vi "PIM System Warning.vi"(6 "Driver Ref (null)":T1, 8 "error in (no error)":errorcluster, 10 "PIM Test Parameters":T2={"Stimulus"={"C1 Pwr dBm"=0.0, "C2 Pwr dBm"=0.0, "Power Units"=enum."dBm", "Meas Type"=enum."Time", "C1 Freq MHz"=0.0, "C2 Freq MHz"=0.0, "Swept Freq Step"=0}, "Measure"={"IM Order"=0, "Direction"=0, "Averaging"=1, "ALC ON?"=TRUE, "Peak Hold?"=TRUE, "Peak last N"=1, "Ref Level dBm"=-100.0, "Ref Units"=enum."dBm", "Num Samples"=1, "Sample units"=enum."Sample(s)", "Update Rate (s)"=0.0, "DUT PORT"=enum."Port 1", "Percent (%)"=100}, "Display"={"Power Scale"={"yRange_min"=0, "yRange_max"=0}, "xRange_span"=5}} {"Stimulus"."Swept Freq Step" items=[".2", ".4", "1.0", "2.0"]; "Measure"."Averaging" items=["None", "Minimum", "Normal", "High", "Maximum"]; "Measure"."Direction" items=["Reverse", "Forward", "Auxiliary"]; "Measure"."IM Order" items=["3rd", "5th", "7th", "9th", "11th", "13th", "15th", "17th", "19th", "21st", "23rd", "25th", "27th", "29th", "31st", "33rd"]}, 11 "TestSetDef":T12={"General"={"ID"=0, "Model"="", "Dual Port?"=FALSE, "Options"="", "Options"={"E"=FALSE, "K"=FALSE, "H"=FALSE, "W"=FALSE, "F"=FALSE}, "Cal File"=path ""}, "Receiver"={"Fstart, MHz"=0.0, "Fstop MHz"=0.0, "Fstep MHz"=0.0, "IF, MHz"=0.0}, "RX Band"={"Fstart, MHz"=0.0, "Fstop MHz"=0.0}, "TX 1"={"Fstart, MHz"=0.0, "Fstop MHz"=0.0, "Pmax, dBm"=0.0, "Pstep, dB"=0.0}, "TX 2"={"Fstart, MHz"=0.0, "Fstop MHz"=0.0, "Pmax, dBm"=0.0, "Pstep, dB"=0.0}, "Low-side?"=TRUE}) -> (2 "Message (\"\")":string="\n\n", 3 "Abort?":bool)   [LabVIEW 2011]
uses:
  BPIMCore/HW IO/Test Set Definition.ctl
  TypeDefs/PIM Test Parameters.ctl
  TypeDefs/PIM Stimulus Parameters.ctl
  BPIMCore/HW IO/PIM Sweep Step Size.ctl
  TypeDefs/PIM Measurement Parameters.ctl
  BPIMCore/HW IO/IMOrder.ctl
  BPIMCore/HW IO/MeasMode.ctl
  BPIMCore/HW IO/HW Averaging.ctl
  TypeDefs/PIM Meas Units.ctl
  BPIMCore/HW IO/DUTport.ctl
  TypeDefs/PIM Display Parameters.ctl
  drivers/PIM/PIM Driver Ref.ctl
  drivers/PIM/PIM Command.ctl
panel:
  in  "B 2":bool
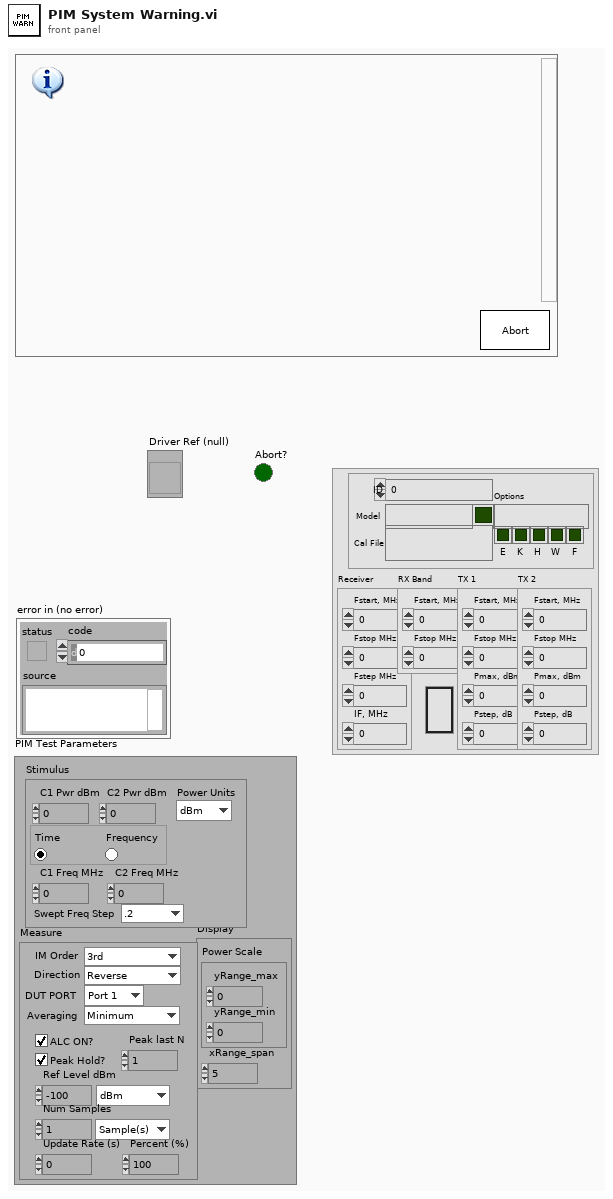
[diagram p1: front panel]
types:
  T1 = typedef "PIM Driver Ref.ctl" = refnum<vi>
  T2 = typedef "PIM Test Parameters.ctl" = cluster{"Stimulus":T3, "Measure":T5, "Display":T11}
  T3 = typedef "PIM Stimulus Parameters.ctl" = cluster{"C1 Pwr dBm":dbl, "C2 Pwr dBm":dbl, "Power Units":enum16{"dBm", "Watts"}, "Meas Type":enum32{"Time", "Frequency"}, "C1 Freq MHz":dbl, "C2 Freq MHz":dbl, "Swept Freq Step":T4}
  T4 = typedef "PIM Sweep Step Size.ctl" = u16
  T5 = typedef "PIM Measurement Parameters.ctl" = cluster{"IM Order":T6, "Direction":T7, "Averaging":T8, "ALC ON?":bool, "Peak Hold?":bool, "Peak last N":u32, "Ref Level dBm":dbl, "Ref Units":enum16{"dBm", "dBc"}, "Num Samples":u32, "Sample units":T9, "Update Rate (s)":dbl, "DUT PORT":T10, "Percent (%)":u8}
  T6 = typedef "IMOrder.ctl" = u8
  T7 = typedef "MeasMode.ctl" = u16
  T8 = typedef "HW Averaging.ctl" = u16
  T9 = typedef "PIM Meas Units.ctl" = enum16{"Sample(s)", "Second(s)", "Sweep(s)"}
  T10 = typedef "DUTport.ctl" = enum16{"Port 1", "Port 2"}
  T11 = typedef "PIM Display Parameters.ctl" = cluster{"Power Scale":cluster{"yRange_min":i32, "yRange_max":i32}, "xRange_span":u32}
  T12 = typedef "Test Set Definition.ctl" = cluster{"General":cluster{"ID":u32, "Model":string, "Dual Port?":bool, "Options":string, "Options":cluster{"E":bool, "K":bool, "H":bool, "W":bool, "F":bool}, "Cal File":path}, "Receiver":cluster{"Fstart, MHz":dbl, "Fstop MHz":dbl, "Fstep MHz":dbl, "IF, MHz":dbl}, "RX Band":cluster{"Fstart, MHz":dbl, "Fstop MHz":dbl}, "TX 1":cluster{"Fstart, MHz":dbl, "Fstop MHz":dbl, "Pmax, dBm":dbl, "Pstep, dB":dbl}, "TX 2":cluster{"Fstart, MHz":dbl, "Fstop MHz":dbl, "Pmax, dBm":dbl, "Pstep, dB":dbl}, "Low-side?":bool}
  T13 = cluster{"Fstart, MHz":dbl, "Fstop MHz":dbl, "Pmax, dBm":dbl, "Fstart, MHz":dbl, "Fstop MHz":dbl, "Pmax, dBm":dbl, "Fstart, MHz":dbl, "Fstop MHz":dbl}
  T14 = cluster{"C1 Freq MHz":dbl, "C1 Pwr dBm":dbl, "C2 Freq MHz":dbl, "C2 Pwr dBm":dbl}
  T15 = cluster{"[0]":string, "[1]":string, "[2]":string, "[3]":string}
  T16 = cluster{"[0]":string, "[1]":string, "[2]":string, "[3]":string, "[4]":string, "[5]":string, "[6]":string, "[7]":string}
  T17 = typedef "PIM Command.ctl" = enum16{"LOAD", "KEEP ALIVE", "VALIDATE", "INITIALIZE", "PRESET", "GET CALIBRATION", "SET STIMULUS", "TOGGLE TX POWER", "SET TX ON", "SET TX OFF", "MEASURE", "UNLOAD"}
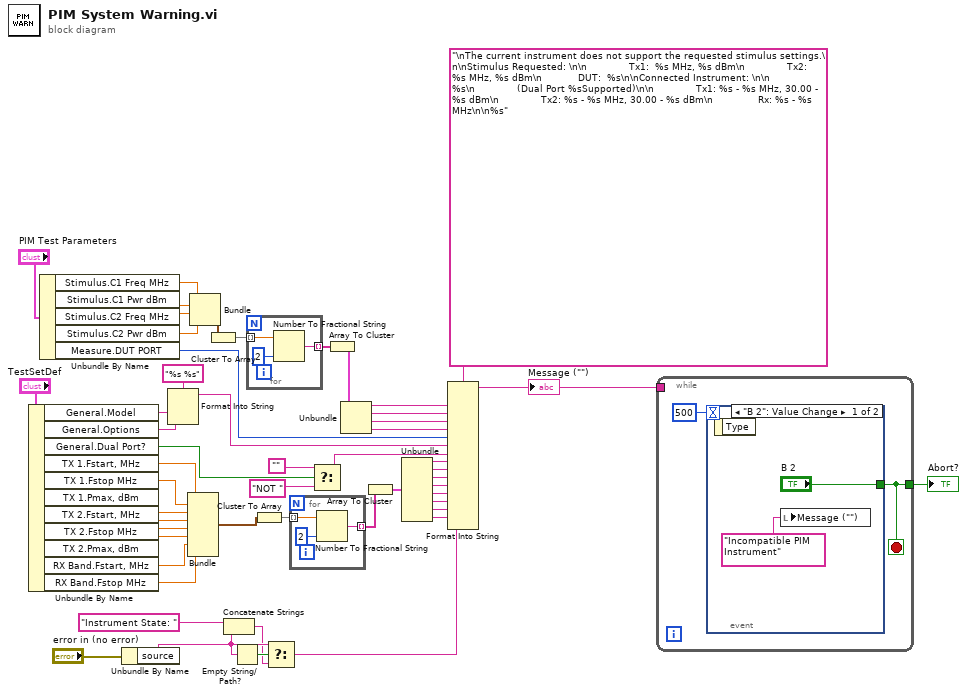
[diagram p0: block diagram]
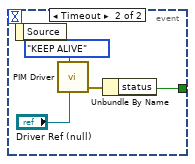
[diagram p2: hidden frame]
diagram:
  n1 = Unbundle By Name("TestSetDef") -> ("General.Model"=w4:string, "General.Options"=w3:string, "General.Dual Port?"=w7:bool, "TX 1.Fstart, MHz"=w46:dbl, "TX 1.Fstop MHz"=w45:dbl, "TX 1.Pmax, dBm"=w44:dbl, "TX 2.Fstart, MHz"=w43:dbl, "TX 2.Fstop MHz"=w42:dbl, "TX 2.Pmax, dBm"=w41:dbl, "RX Band.Fstart, MHz"=w13:dbl, "RX Band.Fstop MHz"=w12:dbl)
  n2 = Unbundle By Name("PIM Test Parameters") -> ("Stimulus.C1 Freq MHz"=w33:dbl, "Stimulus.C1 Pwr dBm"=w32:dbl, "Stimulus.C2 Freq MHz"=w31:dbl, "Stimulus.C2 Pwr dBm"=w30:dbl, "Measure.DUT PORT"=w10:T10)
  n3 = Unbundle By Name("error in (no error)") -> ("source"=w18:string)
  n4 = Format Into String(format string="%s %s", w4, w3) -> (resulting string=w1:string)  [unwired: 2 in, 1 out]
  n5 = Bundle("Fstart, MHz"=w46, "Fstop MHz"=w45, "Pmax, dBm"=w44, "Fstart, MHz"=w43, "Fstop MHz"=w42, "Pmax, dBm"=w41, "Fstart, MHz"=w13, "Fstop MHz"=w12) -> (w47:T13)  [unwired: 1 out]
  n6 = Bundle("C1 Freq MHz"=w33, "C1 Pwr dBm"=w32, "C2 Freq MHz"=w31, "C2 Pwr dBm"=w30) -> (w29:T14)  [unwired: 1 out]
  n7 = Cluster To Array(cluster=w29) -> (array=w28:dbl[])
  n8 = Concatenate Strings("Instrument State: " ("string"), w18) -> (w17:string)
  n9 = Empty String/Path?(string/path=w18) -> (empty?=w20:bool)
  n10 = for {
    tunnel: w28 -> [w55] mode=indexing
    tunnel: [w53] -> w27 mode=indexing
    n11 = Number To Fractional String(number=w55, precision (6)=i16 2) -> (F-format string=w53:string)  [unwired: 2 out]
  }
  n12 = Cluster To Array(cluster=w47) -> (array=w48:dbl[])
  n13 = Select(t=w18, s=w20, f=w17) -> (s? t:f=w16:string)
  n14 = for {
    tunnel: w48 -> [w58] mode=indexing
    tunnel: [w56] -> w50 mode=indexing
    n15 = Number To Fractional String(number=w58, precision (6)=i16 2) -> (F-format string=w56:string)  [unwired: 2 out]
  }
  n16 = Select(t="", s=w7, f="NOT " ("string")) -> (s? t:f=w5:string)
  n17 = Array To Cluster(array=w27) -> (cluster=w26:T15)
  n18 = Unbundle(w26) -> ("[0]"=w22:string, "[1]"=w23:string, "[2]"=w24:string, "[3]"=w25:string)
  n19 = Array To Cluster(array=w50) -> (cluster=w49:T16)
  n20 = Unbundle(w49) -> ("[0]"=w40:string, "[1]"=w39:string, "[2]"=w38:string, "[3]"=w37:string, "[4]"=w36:string, "[5]"=w35:string, "[6]"=w15:string, "[7]"=w14:string)
  n21 = Format Into String(format string="\nThe current instrument does not support the requested stimulus settings.\n\nStimulus Requested: \n\n              Tx1:  %s MHz, %s dBm\n              Tx2:  %s MHz, %s dBm\n            DUT:  %s\n\nConnected Instrument: \n\n              %s\n              (Dual Port %sSupported)\n\n              Tx1: %s - %s MHz, 30.00 - %s dBm\n              Tx2: %s - %s MHz, 30.00 - %s dBm\n               Rx: %s - %s MHz\n\n%s", w22, w23, w24, w25, w10, w1, w5, w40, w39, w38, w37, w36, w35, w15, w14, w16) -> (resulting string=w6:string)  [unwired: 2 in, 1 out]
  "Message (\"\")" <- w6
  n22 = while {
    tunnel: [w60] -> w52
    tunnel: w6 -> [_]
    stop <- w60 stop-if-true
    n23 = event shown="[0] \"B 2\": Value Change" {
      selector: _ -> [_ _]
      dyn-events: _ -> [_ _]
      timeout: 500 -> [_ _]
      tunnel: ["B 2" w63] -> w60
      event "B 2": Value Change {
        n24 = event-data() -> ()  [unwired: 2 out]
        n25 = local write "Message (\"\")"("Incompatible PIM Instrument" ("Message (\"\")")) -> ()
      }
      event Timeout {
        n26 = event-data() -> ()  [unwired: 2 out]
        n27 = call "PIM Driver.vi"("Driver Ref (null)"="Driver Ref (null)", "PIM Command"=PIM_Command."KEEP ALIVE") -> ("error out"=w64:errorcluster)  [unwired: 3 in, 6 out]
        n28 = Unbundle By Name(w64) -> ("status"=w63:bool)
      }
    }
  }
  "Abort?" <- w52
